vi "Start Series.vi"(8 "error in":errorcluster, 11 "Host MSS Test Actor in":refnum<class "Host MSS Test Actor.lvclass">) -> (0 "error out":errorcluster, 3 "Host MSS Test Actor out":refnum<class "Host MSS Test Actor.lvclass">)   [LabVIEW 2023, in "Host MSS Test Actor.lvlib" / "Host MSS Test Actor.lvclass"]
uses:
  Host MSS Test Actor.lvclass
  Host MSS Test Actor.lvclass/Host MSS Test Actor.ctl
  Series/Series Base/Series Base.lvclass
  Task/Task Actor/ITask Actor/ITask Actor Messages/Do Msg/Do Msg.lvclass
  <vilib>/ErrorRing/Error Ring.xnode
  <vilib>/Utility/error.llb/Error Cluster From Error Code.vi
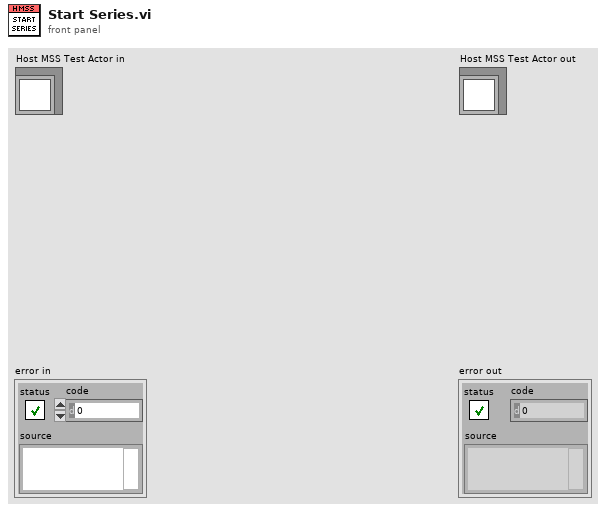
[diagram p1: front panel]
types:
  T1 = map{string, refnum<class "Message Enqueuer.lvclass">}
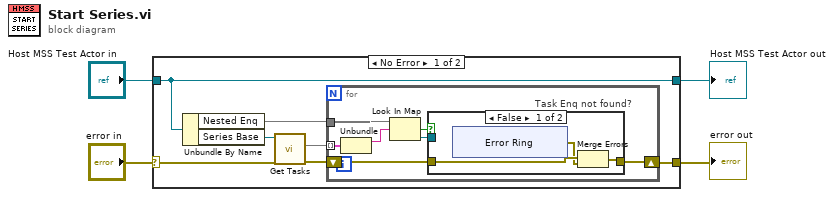
[diagram p0: block diagram]
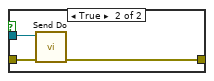
[diagram p2: hidden frame]
diagram:
  n1 = case shown="No Error" "error in" {
    selector: "error in" -> [w7 w31]
    tunnel: "Host MSS Test Actor in" -> [w10 w30]
    tunnel: [w10 w30] -> w1
    tunnel: [w11 w31] -> w2
    frame No Error {
      n2 = Unbundle By Name(w10) -> ("Nested Enq"=w9:T1, "Series Base"=w8:refnum<class "Series Base.lvclass">)
      n3 = call "Get Tasks.vi"("error in (no error)"=w7, "HAL GOOP4:Series Base in"=w8) -> ("error out"=w6:errorcluster, "Tasks"=w5:map{string, refnum<class "Task Base.lvclass">})  [unwired: 7 in, 1 out]
      n4 = for {
        tunnel: w9 -> [w17]
        shift-right: [w12] -> w11
        shift-left: w6 -> [w14]
        tunnel: w5 -> [w18] mode=indexing
        n5 = Unbundle(w18) -> (w16:string)  [unwired: 1 out]
        n6 = Look In Map(map=w17, key=w16) -> (key not found?=w15:bool, value=w13:refnum<class "Message Enqueuer.lvclass">)  [unwired: 1 in]
        n7 = case "Task Enq not found?" shown="False" w15 {
          tunnel: w14 -> [w20 w29]
          tunnel: w13 -> [_ w28]
          tunnel: [w21 w27] -> w12
          frame False {
            n8 = xnode "Error Ring"() -> ("error out"=w19:errorcluster)
            n9 = Merge Errors(w20, w19) -> (w21:errorcluster)
          }
          frame True {
            n10 = call "Send Do.vi"("error in (no error)"=w29, "Message Enqueuer"=w28) -> ("error out"=w27:errorcluster)  [unwired: 8 in, 1 out]
          }
        }
      }
    }
    frame Error {
    }
  }
  "error out" <- w2
  "Host MSS Test Actor out" <- w1
